vi "CAEN_HV_subvi_read.vi"(5 "handle HV1":i32, 6 "handle HV2":i32, 7 "error in (no error)":errorcluster) -> (0 "handle HV1 out":i32, 1 "HV":sgl[](array[numeric]), 2 "Current":sgl[](array[numeric]), 3 "error out":errorcluster, 4 "handle HV2 out":i32)   [LabVIEW 2012]
uses:
  CAEN/labview/CAENHVWrapper/CAENHVWrapper.lvlib
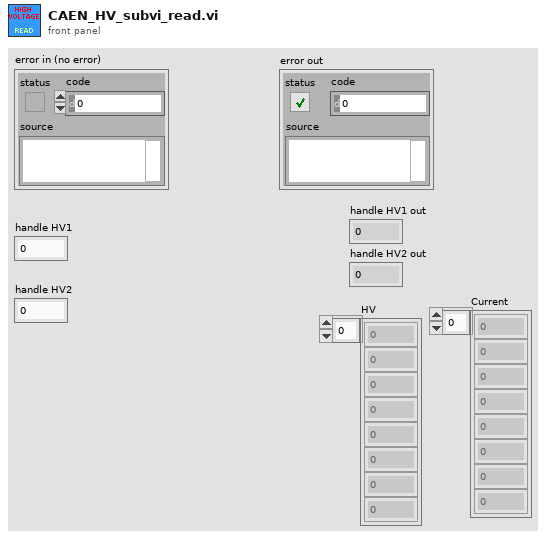
[diagram p1: front panel]
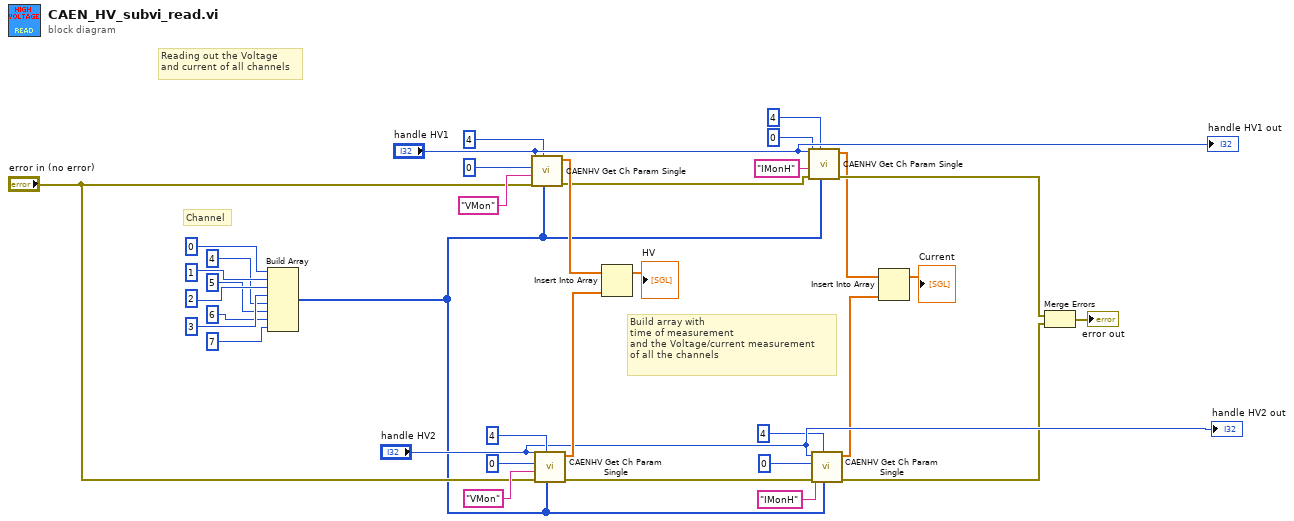
[diagram p0: block diagram]
diagram:
  # "Build array with \ntime of measurement \nand the Voltage/current measurement \nof all the channels"
  # "Channel"
  # "Reading out the Voltage\nand current of all channels"
  n1 = Build Array(0, 1, 2, 3, 4, 5, 6, 7) -> (w1:i32[])
  n2 = call "CAENHV Get Ch Param Single.vi"("ChList"=w1, "ChNum (1)"=u16 4, "error in (no error)"="error in (no error)", "ParName"="VMon", "slot"=u16 0, "handle"="handle HV1") -> ("error out"=w19:errorcluster, "ParValList"=w23:sgl[])  [unwired: 4 in]
  n3 = call "CAENHV Get Ch Param Single.vi"("ChList"=w1, "ChNum (1)"=u16 4, "error in (no error)"="error in (no error)", "ParName"="VMon", "slot"=u16 0, "handle"="handle HV2") -> ("error out"=w9:errorcluster, "ParValList"=w24:sgl[])  [unwired: 4 in]
  n4 = Insert Into Array(array=w23, new element=w24) -> (→"HV":sgl[])  [unwired: 1 in]
  n5 = call "CAENHV Get Ch Param Single.vi"("ChList"=w1, "ChNum (1)"=u16 4, "error in (no error)"=w19, "ParName"="IMonH", "slot"=u16 0, "handle"="handle HV1") -> ("error out"=w18:errorcluster, "ParValList"=w5:sgl[])  [unwired: 4 in]
  n6 = call "CAENHV Get Ch Param Single.vi"("ChList"=w1, "ChNum (1)"=u16 4, "error in (no error)"=w9, "ParName"="IMonH", "slot"=u16 0, "handle"="handle HV2") -> ("error out"=w8:errorcluster, "ParValList"=w6:sgl[])  [unwired: 4 in]
  n7 = Insert Into Array(array=w5, new element=w6) -> (→"Current":sgl[])  [unwired: 1 in]
  n8 = Merge Errors(w18, w8) -> (→"error out":errorcluster)
  "handle HV1 out" <- "handle HV1"
  "handle HV2 out" <- "handle HV2"
